vi "Heartbeat Producer.vi"(8 "error in":errorcluster, 10 "Interval":i32 format="%d ms", 11 "CANopen Master in":refnum<class "CANopen Master.lvclass">) -> ()   [LabVIEW 2024, in "CANopen Master.lvlib" / "CANopen Master.lvclass"]
uses:
  CANopen Master.lvclass
  CANopen Master.lvclass/CANopen Master.ctl
  CANopen Message/CANopen Message.lvclass
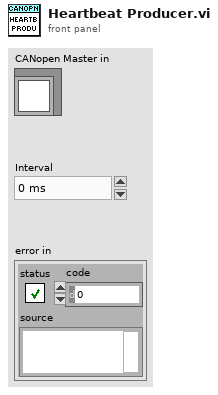
[diagram p1: front panel]
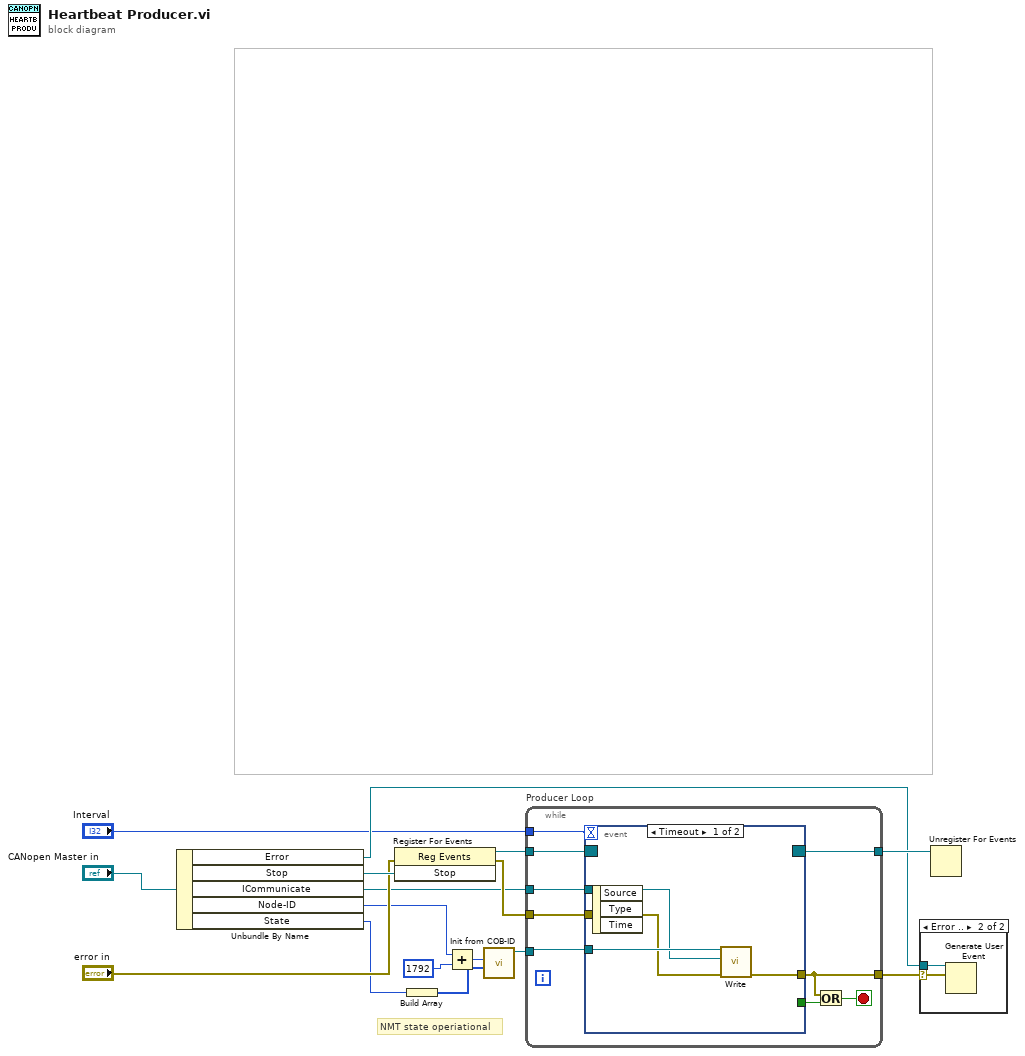
[diagram p0: block diagram]
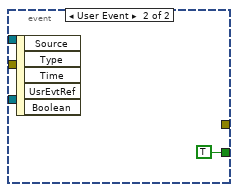
[diagram p2: hidden frame]
diagram:
  # "NMT state operiational"
  n1 = Unbundle By Name("CANopen Master in") -> ("Error"=w9:refnum<user-event>, "Stop"=w13:refnum<user-event>, "ICommunicate"=w8:refnum<class "ICommunicate.lvclass">, "Node-ID"=w4:u8, "State"=w2:u16)
  n2 = register-events(error in="error in", w13) -> (reference out=w14:refnum<event-registration>, error out=w11:errorcluster)  [unwired: 1 in]
  n3 = Build Array(w2) -> (w1:u16[])
  n4 = Add(x=w4, y=u32 1792 ("COB-ID")) -> (x+y=w6:u32)
  n5 = call "Init from COB-ID.vi"("Data"=w1, "COB-ID"=w6) -> ("CANopen Message out"=w5:refnum<class "CANopen Message.lvclass">)  [unwired: 9 in]
  n6 = while "Producer Loop" {
    tunnel: [w23] -> w16
    tunnel: w14 -> [w22]
    tunnel: w11 -> [w25]
    tunnel: [w20] -> w10
    tunnel: w8 -> [w19]
    tunnel: "Interval" -> [w18]
    tunnel: w5 -> [w17]
    stop <- w24 stop-if-true
    n7 = event shown="[0] Timeout" {
      selector: w22 -> [_ _]
      dyn-events: [_ _] -> w23
      timeout: w18 -> [_ _]
      tunnel: w25 -> [w27 _]
      tunnel: [w26 _] -> w20
      tunnel: [_ TRUE] -> w21
      tunnel: w19 -> [w28 _]
      tunnel: w17 -> [w29 _]
      event Timeout {
        n8 = event-data() -> ()  [unwired: 1 in, 3 out]
        n9 = call "Write.vi"("error in"=w27, "ICommunicate"=w28, "CANopen Message in"=w29) -> ("error out"=w26:errorcluster)  [unwired: 7 in, 1 out]
      }
      event User Event {
        n10 = event-data() -> ()  [unwired: 1 in, 5 out]
      }
    }
    n11 = Or(x=w20, y=w21) -> (x .or. y?=w24:bool)
  }
  n12 = case shown="Error .." w10 {
    selector: w10 -> [_ w31]
    tunnel: w9 -> [_ w32]
    frame No Error {
    }
    frame Error {
      n13 = Generate User Event(user event=w32, event data cluster=w31) -> ()  [unwired: 2 in, 2 out]
    }
  }
  n14 = Unregister For Events(event registration refnum=w16) -> ()  [unwired: 1 in, 1 out]
